vi "Joud_signal_generation_Test.vi"(8 "error in":errorcluster) -> (0 "error out":errorcluster, 3 "task out":refnum<k21>)   [LabVIEW 2020]
uses:
  <vilib>/DAQmx/create/channels.llb/DAQmx Create Channel (AI-Acceleration-Accelerometer).vi
  <vilib>/DAQmx/configure/timing.llb/DAQmx Timing (Sample Clock).vi
  <resource>/objmgr/daqmx.rc
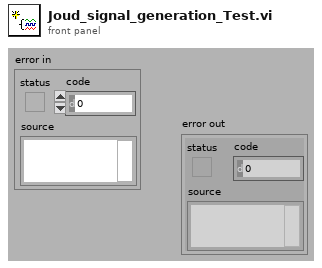
[diagram p1: front panel]
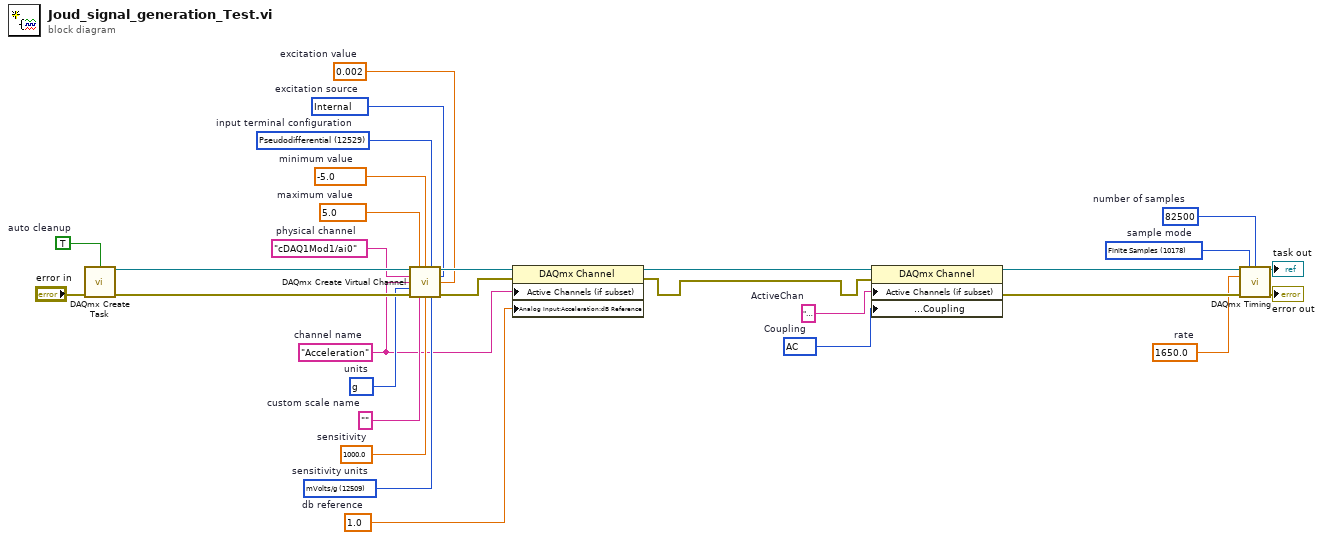
[diagram p0: block diagram]
diagram:
  w1 = 10178 items=["Finite Samples"=10178, "Continuous Samples"=10123, "Hardware Timed Single Point"=12522]  # sample mode
  w2 = 82500  # number of samples
  w3 = 1650.0  # rate
  w9 = 10045 items=["AC"=10045, "DC"=10050, "GND"=10066]  # Coupling
  w10 = "Acceleration"  # ActiveChan
  w12 = 1.0  # db reference
  w15 = 10186 items=["g"=10186, "m/s^2"=12470, "From Custom Scale"=10065]  # units
  w16 = 12529 items=["default"=-1, "RSE"=10083, "NRSE"=10078, "Differential"=10106, "Pseudodifferential"=12529]  # input terminal configuration
  w17 = 10200 items=["Internal"=10200, "External"=10167, "None"=10230]  # excitation source
  w18 = 0.002  # excitation value
  w19 = 12509 items=["mVolts/g"=12509, "Volts/g"=12510]  # sensitivity units
  w20 = 1000.0  # sensitivity
  w11 = "Acceleration"  # channel name
  w22 = ""  # custom scale name
  w23 = -5.0  # minimum value
  w24 = 5.0  # maximum value
  w25 = "cDAQ1Mod1/ai0"  # physical channel
  w27 = TRUE  # auto cleanup
  n1 = call <vilib>:"DAQmx Create Task.vi"("auto cleanup"=w27, "error in"="error in") -> ("task out"=w26:refnum<k21>, "error out"=w28:errorcluster)  [unwired: 12 in]
  n2 = call-poly <vilib>:"DAQmx Create Virtual Channel.vi"("task in"=w26, "maximum value"=w24, "minimum value"=w23, "input terminal configuration"=w16, "physical channels"=w25, "current excitation source"=w17, "name to assign"=w11, "current excitation value"=w18, "units"=w15, "error in"=w28, "custom scale name"=w22, "sensitivity"=w20, "sensitivity units"=w19) -> ("task out"=w21:refnum<k21>, "error out"=w14:errorcluster)  [unwired: 1 in]
  n3 = property class="DAQmx Channel"(reference=w21, error in=w14, "Active Channels (if subset)"=w11, "Analog Input:Acceleration:dB Reference"=w12) -> (reference out=w7:refnum<k21>, error out=w13:errorcluster)
  n4 = property class="DAQmx Channel"(reference=w7, error in=w13, "Active Channels (if subset)"=w10, "Analog Input:General Properties:Input Configuration:Coupling"=w9) -> (reference out=w4:refnum<k21>, error out=w8:errorcluster)
  n5 = call-poly <vilib>:"DAQmx Timing.vi"("task/channels in"=w4, "sample mode"=w1, "samples per channel"=w2, "rate"=w3, "error in"=w8) -> ("task out"=→"task out":refnum<k21>, "error out"=→"error out":errorcluster)  [unwired: 9 in]
